vi "Logarithmic Sweep.vi"(0 "Sweep Parameters":T1={"Start"=1.0, "End"=10.0, "Samples"=128} {"End" format="%#_13g"; "Start" format="%#_13g"}, 11 "error in (no error)":errorcluster) -> (4 "Ramp Pattern":dbl[](array[numeric]), 15 "error out":errorcluster)   [LabVIEW 2020]
doc: "Lograthmic sweep performs a Logarthmic sweep for N Samples from start to end. This VI also handles negative and zero values in the input sweep parameters where the output will be returned as empty array."
uses:
  Sweep Parameters.ctl
  <vilib>/Analysis/1siggen.llb/Ramp Pattern by Samples.vi
  <vilib>/Analysis/NI_AALBase.lvlib
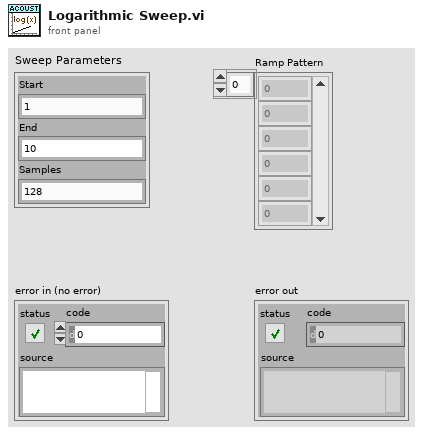
[diagram p1: front panel]
types:
  T1 = typedef "Sweep Parameters.ctl" = cluster{"Start":dbl, "End":dbl, "Samples":i32}
  T2 = cluster{"Start":bool, "End":bool, "Samples":bool}
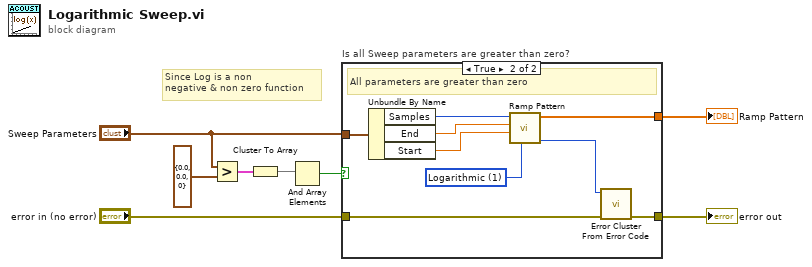
[diagram p0: block diagram]
diagram:
  # "Since Log is a non\nnegative & non zero function"
  n1 = Greater?(x="Sweep Parameters", y=T1 {"Start"=0.0, "End"=0.0, "Samples"=0} ("Sweep Parameters")) -> (0:w3:T2)
  n2 = Cluster To Array(cluster=w3) -> (array=w2:bool[])
  n3 = And Array Elements(Boolean array=w2) -> (logical AND=w1:bool)
  n4 = case "Is all Sweep parameters are greater than zero?" shown="True" w1 {
    tunnel: "error in (no error)" -> [w9 w17]
    tunnel: [_ w13] -> w7
    tunnel: [w9 w12] -> w6
    tunnel: "Sweep Parameters" -> [_ w10]
    frame False {
      # "One or more parameters are lesser are equal to zero"
    }
    frame True {
      w18 = u16 1 items=["Linear", "Logarithmic"] ("type")
      # "All parameters are greater than zero"
      n5 = Unbundle By Name(w10) -> ("Samples"=w16:i32, "End"=w15:dbl, "Start"=w14:dbl)
      n6 = call-poly <vilib>:"Ramp Pattern.vi"("type"=w18, "start"=w14, "end"=w15, "samples"=w16) -> ("error"=w11:i32, "Ramp Pattern"=w13:dbl[])  [unwired: 6 in]
      n7 = call <vilib>:"Error Cluster From Error Code.vi"("error in (no error)"=w17, "error code (0)"=w11) -> ("error out"=w12:errorcluster)  [unwired: 7 in]
    }
  }
  "error out" <- w6
  "Ramp Pattern" <- w7
